vi "Disconnect.vi"(8 "error in (no error)":errorcluster, 11 "NI Vision Camera Device in":refnum<class "NI Vision Camera Device.lvclass">) -> (0 "error out":errorcluster, 3 "NI Vision Camera Device out":refnum<class "NI Vision Camera Device.lvclass">)   [LabVIEW 2014, in "NI Vision Camera Device.lvclass"]
uses:
  NI Vision Camera Device.lvclass
  NI Vision Camera Device.lvclass/NI Vision Camera Device.ctl
  <vilib>/vision/driver/NI_Vision_Acquisition_Software.lvlib
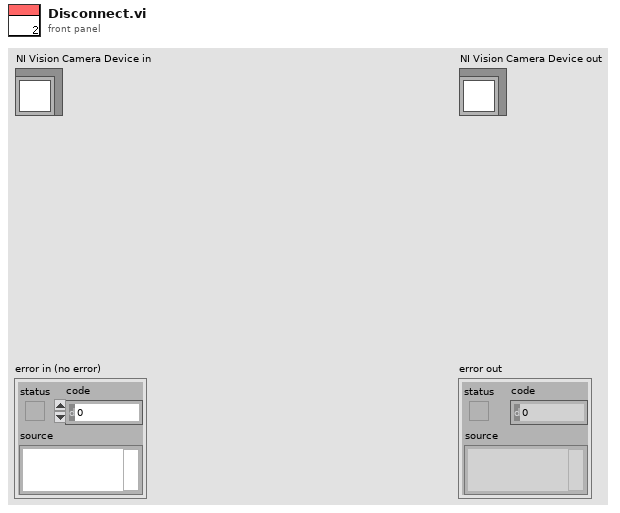
[diagram p1: front panel]
types:
  T1 = typedef "IMAQdx.ctl" = refnum<k21>
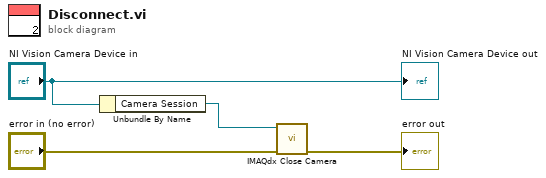
[diagram p0: block diagram]
diagram:
  n1 = Unbundle By Name("NI Vision Camera Device in") -> ("Camera Session"=w3:T1)
  n2 = call <vilib>:"IMAQdx Close Camera.vi"("error in"="error in (no error)", "Session In"=w3) -> ("error out"=→"error out":errorcluster)  [unwired: 9 in]
  "NI Vision Camera Device out" <- "NI Vision Camera Device in"
